vi "CRYConvert Unicode to ASCII.vi"(4 "Unicode":string, 5 "Code Page":u32(ring) items=["System default"=0, "Latin-1"=1252, "Japanese"=932, "Korean"=949, "Chinese simplified"=936, "Chinese traditional"=950, "Central Europe"=1250, "Cyrillic"=1251, "Greek"=1253, "Turkish"=1254, "Hebrew"=1255, "Arabic"=1256, "Baltic"=1257, "Thai"=874, "Vietnamese"=783, "UTF8"=65001, "UTF-7"=65000]) -> (1 "ASCII":string)   [LabVIEW 2013]
uses:
  Kernel32.DLL
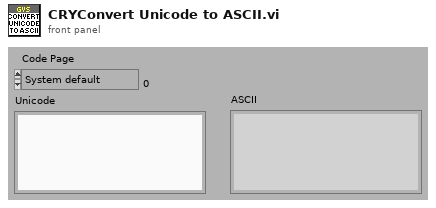
[diagram p1: front panel]
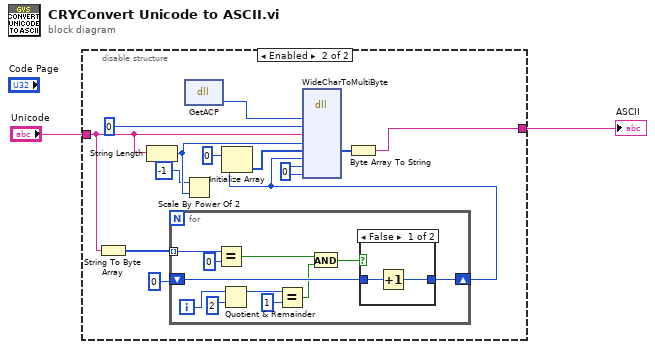
[diagram p0: block diagram]
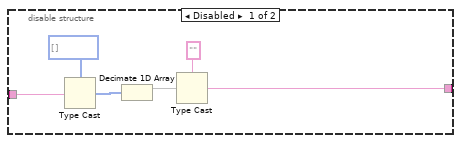
[diagram p2: hidden frame]
diagram:
  n1 = disable-structure shown="Enabled" {
    disable-tunnel: "Unicode" -> [w8 w11]
    disable-tunnel: [w5 w16] -> w1
    frame Disabled {
      n2 = Type Cast(type=u8[] [], x=w8) -> (*(type *) &x=w4:u8[])
      n3 = Decimate 1D Array(w4) -> (w3:u8[])  [unwired: 1 out]
      n4 = Type Cast(type="", x=w3) -> (*(type *) &x=w5:string)
    }
    frame Enabled {
      w13 = u32 0
      n5 = String To Byte Array(string=w11) -> (unsigned byte array=w10:u8[])
      n6 = String Length(string=w11) -> (length=w15:i32)
      n7 = for {
        tunnel: w10 -> [w32] mode=indexing
        shift-right: [w30] -> w9
        shift-left: 0 -> [w29]
        i -> [w28]
        n8 = Equal?(x=w32, y=u8 0) -> (x = y?=w26:bool)
        n9 = Quotient & Remainder(x=w28, y=2) -> (x-y*floor(x/y)=w24:i32)  [unwired: 1 out]
        n10 = Equal?(x=w24, y=1) -> (x = y?=w22:bool)
        n11 = And(x=w26, y=w22) -> (x .and. y?=w25:bool)
        n12 = case shown="False" w25 {
          tunnel: w29 -> [w33 w35]
          tunnel: [w34 w35] -> w30
          frame False {
            n13 = Increment(x=w33) -> (x+1=w34:i32)
          }
          frame True {
          }
        }
      }
      n14 = Scale By Power Of 2(n=-1, x=w15) -> ()  [unwired: 1 out]
      n15 = dll-call lib="kernel32.dll" fn="GetACP" label="GetACP()"() -> (w21:u32)  [unwired: 3 in, 2 out]
      n16 = Initialize Array(u8 0, w9) -> (w19:u8[])
      n17 = dll-call lib="Kernel32.DLL" fn="WideCharToMultiByte"("codePage"=w21, "dwFlags"=u32 0, "lpWideCharStr"=w11, "cchWideChar"=w15, "lpMultiByteStr"=w19, "cbMultiByte"=w9, "lpDefaultChar"=w13, "lpUsedDefaultChar"=w13) -> ("lpMultiByteStr"=w20:u8[])  [unwired: 10 in, 3 out]
      n18 = Byte Array To String(unsigned byte array=w20) -> (string=w16:string)
    }
  }
  "ASCII" <- w1
